vi "calc_gettimestamp.vi"(8 "error in (no error)":errorcluster) -> (0 "error out":errorcluster, 3 "Timestamp":timestamp)   [LabVIEW 2018]
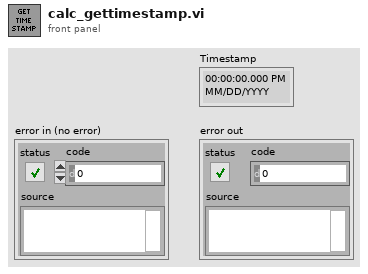
[diagram p1: front panel]
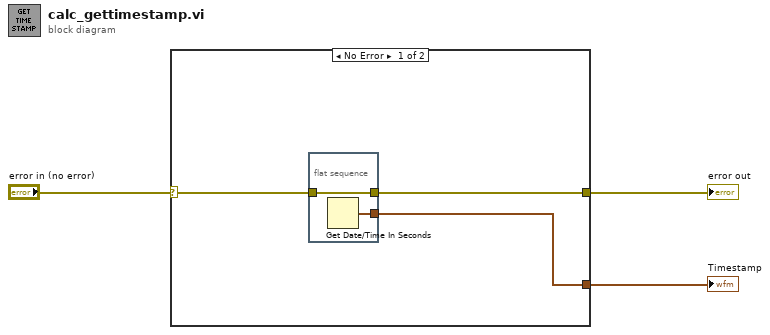
[diagram p0: block diagram]
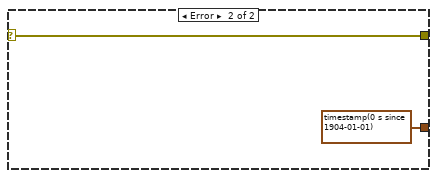
[diagram p2: hidden frame]
diagram:
  n1 = case shown="No Error" "error in (no error)" {
    selector: "error in (no error)" -> [w4 w10]
    tunnel: [w6 timestamp(0 s since 1904-01-01) ("seconds since 1Jan1904")] -> w3
    tunnel: [w5 w10] -> w2
    frame No Error {
      n2 = flat-sequence {
        tunnel: w4 -> [w8]
        tunnel: [w8] -> w5
        tunnel: [w7] -> w6
        frame #0 {
          n3 = Get Date/Time In Seconds() -> (seconds since 1Jan1904=w7:timestamp)
        }
      }
    }
    frame Error {
    }
  }
  "error out" <- w2
  "Timestamp" <- w3
